vi "Untitled4.vi"() -> ()   [LabVIEW 2024]
uses:
  CANopen Master/CANopen Master.lvclass
  HAL/HAL/Devices/CAN Interfaces/PCAN/PCAN.lvclass
  D:/git/HAL/HAL/Configurations/CFG Base/CFG Base.lvclass
  D:/git/HAL/HAL/Protocols/ICAN/ICAN.lvclass
  CANopen Master/CANopen Master.lvclass/CANopen Master.ctl
  HAL/HAL/Configurations/CFG Base/CFG Base.lvclass
panel:
  in  "Discover Button":bool
  out "Success? DL":bool
  in  "Value":u16
  in  "Multiplexer DL":cluster{"Index":u16, "Sub-Index":u8} {"Index" format="%.0x"}
  in  "Download Button":bool
  in  "Node-ID DL":u8
  out "Available Nodes":map{u8, u8}(c390)
  out "Success? UL":bool
  out "Data UL":u8[](array[numeric]) format="%.0x"
  in  "Node-ID UPL":u8
  in  "Multiplexer":cluster{"Index":u16, "Sub-Index":u8} {"Index" format="%.0x"}
  in  "Upload Button":bool
  out "Emergency?":bool[](array[boolean])
  out "Nodes":u8[](array[numeric])
  in  "stop":bool
  out "Timed Outs?":bool[](array[boolean])
  out "Node-IDs":u8[](array[numeric])
  out "error out":errorcluster
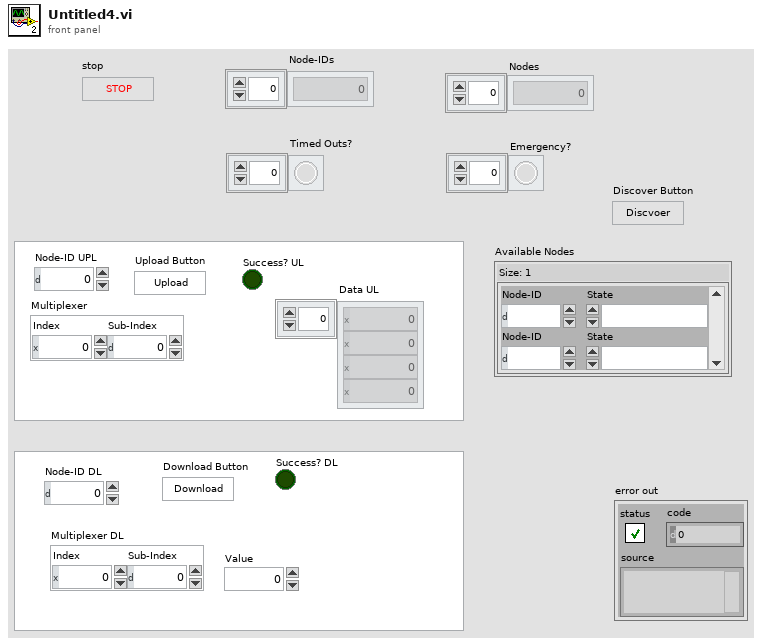
[diagram p1: front panel]
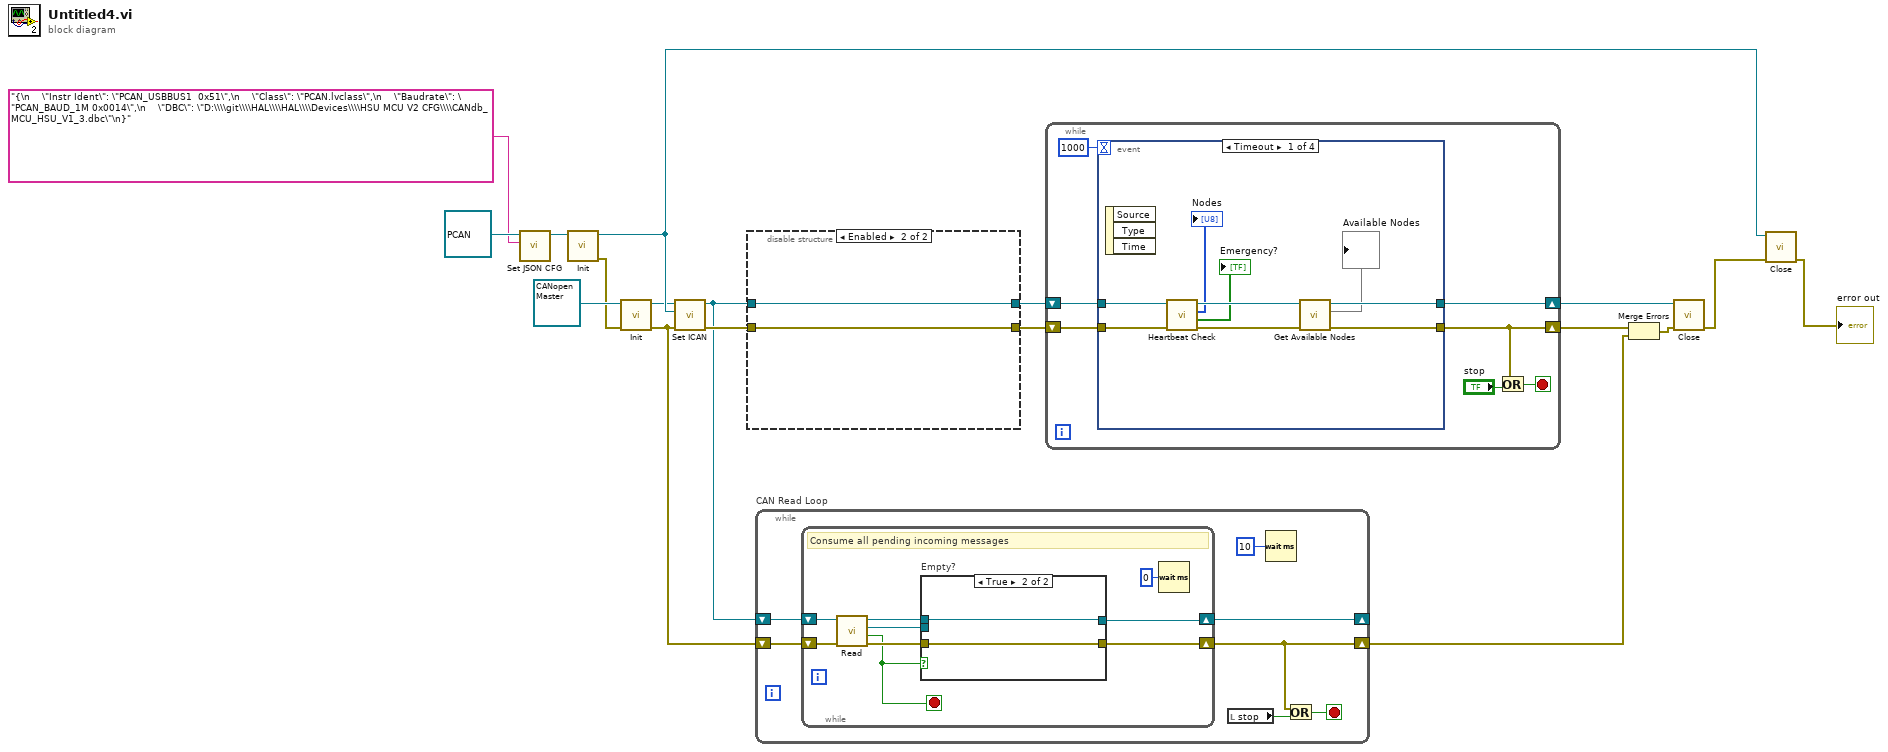
[diagram p0: block diagram]
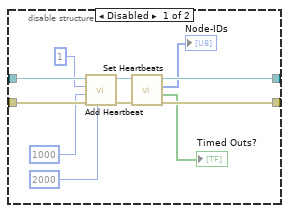
[diagram p2: hidden frame]
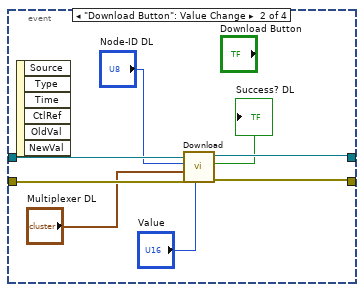
[diagram p3: hidden frame]
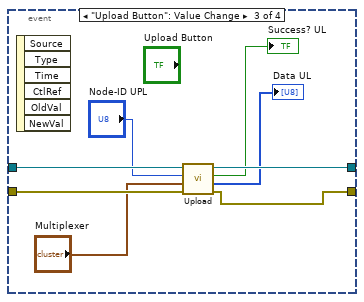
[diagram p4: hidden frame]
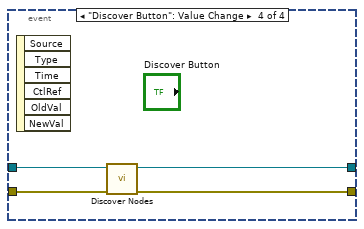
[diagram p5: hidden frame]
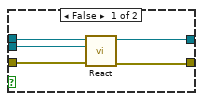
[diagram p6: hidden frame]
diagram:
  n1 = call "Set JSON CFG.vi"("<JSON>CFG"="{\n    \"Instr Ident\": \"PCAN_USBBUS1  0x51\",\n    \"Class\": \"PCAN.lvclass\",\n    \"Baudrate\": \"PCAN_BAUD_1M 0x0014\",\n    \"DBC\": \"D:\\\\git\\\\HAL\\\\HAL\\\\Devices\\\\HSU MCU V2 CFG\\\\CANdb_MCU_HSU_V1_3.dbc\"\n}", "CFG Base in"=refnum<class "PCAN.lvclass"> refnum ("PCAN.lvclass")) -> ("CFG Base out"=w15:refnum<class "PCAN.lvclass">)  [unwired: 9 in]
  n2 = call-dynamic "Init.vi"("PCAN in"=w15) -> ("error out"=w13:errorcluster, "PCAN out"=w12:refnum<class "PCAN.lvclass">)  [unwired: 9 in]
  n3 = call "Init.vi"("error in"=w13, "CANopen Master in"=refnum<class "CANopen Master.lvclass"> refnum ("CANopen Master.lvlib:CANopen Master")) -> ("error out"=w8:errorcluster, "CANopen Master out"=w9:refnum<class "CANopen Master.lvclass">)  [unwired: 8 in]
  n4 = call "Set ICAN.vi"("ICAN"=w12, "CANopen Master in"=w9) -> ("CANopen Master out"=w7:refnum<class "CANopen Master.lvclass">)  [unwired: 9 in]
  n5 = disable-structure shown="Enabled" {
    disable-tunnel: w8 -> [w28 w29]
    disable-tunnel: w7 -> [w27 w30]
    disable-tunnel: [w26 w30] -> w4
    disable-tunnel: [w25 w29] -> w3
    frame Disabled {
      n6 = call "Add Heartbeat.vi"("Timeout"=u16 2000, "error in"=w28, "Period"=u16 1000, "Node-ID"=u8 1, "CANopen Master in"=w27) -> ("error out"=w21:errorcluster, "CANopen Master out"=w20:refnum<class "CANopen Master.lvclass">)  [unwired: 5 in]
      n7 = call "Set Heartbeats.vi"("error in"=w21, "CANopen Master in"=w20) -> ("error out"=w25:errorcluster, "Timed Outs?"=→"Timed Outs?":bool[], "Node-IDs"=→"Node-IDs":u8[], "CANopen Master out"=w26:refnum<class "CANopen Master.lvclass">)  [unwired: 6 in]
    }
    frame Enabled {
    }
  }
  n8 = while "CAN Read Loop" {
    shift-right: [w34] -> w5
    shift-left: w8 -> [w37]
    shift-right: [w33] -> _
    shift-left: w7 -> [w36]
    stop <- w35 stop-if-true
    n9 = while {
      shift-right: [w43] -> w34
      shift-left: w37 -> [w46]
      shift-right: [w39] -> w33
      shift-left: w36 -> [w45]
      stop <- w38 stop-if-true
      # "Consume all pending incoming messages"
      n10 = call "Read.vi"("error in"=w46, "CANopen Master in"=w45) -> ("error out"=w42:errorcluster, "Empty?"=w38:bool, "CANopen Message out"=w44:refnum<class "CANopen Message.lvclass">, "CANopen Master out"=w40:refnum<class "CANopen Master.lvclass">)  [unwired: 6 in]
      n11 = case "Empty?" shown="True" w38 {
        tunnel: w44 -> [w47 _]
        tunnel: [w50 w53] -> w43
        tunnel: w42 -> [w51 w53]
        tunnel: w40 -> [w49 w52]
        tunnel: [w48 w52] -> w39
        frame False {
          n12 = call "React.vi"("error in"=w51, "CANopen Message"=w47, "CANopen Master in"=w49) -> ("error out"=w50:errorcluster, "CANopen Master out"=w48:refnum<class "CANopen Master.lvclass">)  [unwired: 7 in]
        }
        frame True {
        }
      }
      n13 = Wait (ms)(milliseconds to wait=u32 0) -> ()  [unwired: 1 out]
    }
    n14 = local read "stop"() -> (w31:bool)
    n15 = Wait (ms)(milliseconds to wait=10) -> ()  [unwired: 1 out]
    n16 = Or(x=w34, y=w31) -> (x .or. y?=w35:bool)
  }
  n17 = while {
    shift-right: [w57] -> w1
    shift-left: w4 -> [w59]
    shift-right: [w56] -> w2
    shift-left: w3 -> [w58]
    stop <- w55 stop-if-true
    n18 = event shown="[0] Timeout" {
      selector: _ -> [_ _ _ _]
      dyn-events: _ -> [_ _ _ _]
      timeout: 1000 -> [_ _ _ _]
      tunnel: w59 -> [w67 w75 w84 w87]
      tunnel: w58 -> [w68 w76 w83 w88]
      tunnel: [w66 w74 w80 w86] -> w56
      tunnel: [w62 w73 w79 w85] -> w57
      event Timeout {
        n19 = event-data() -> ()  [unwired: 1 in, 3 out]
        n20 = call "Heartbeat Check.vi"("error in"=w68, "CANopen Master in"=w67) -> ("error out"=w66:errorcluster, "Emergency?"=→"Emergency?":bool[], "Nodes"=→"Nodes":u8[], "CANopen Master out"=w65:refnum<class "CANopen Master.lvclass">)  [unwired: 6 in]
        n21 = call "Get Available Nodes.vi"("CANopen Master in"=w65) -> ("Nodes"=→"Available Nodes":map{u8, u8}, "CANopen Master out"=w62:refnum<class "CANopen Master.lvclass">)  [unwired: 8 in, 1 out]
      }
      event "Download Button": Value Change {
        n22 = event-data() -> ()  [unwired: 1 in, 6 out]
        n23 = call "Download.vi"("Value"="Value", "error in"=w76, "Multiplexer"="Multiplexer DL", "Node-ID"="Node-ID DL", "CANopen Master in"=w75) -> ("error out"=w74:errorcluster, "Success?"=→"Success? DL":bool, "CANopen Master out"=w73:refnum<class "CANopen Master.lvclass">)  [unwired: 4 in]
      }
      event "Upload Button": Value Change {
        n24 = event-data() -> ()  [unwired: 1 in, 6 out]
        n25 = call "Upload.vi"("error in"=w83, "Multiplexer"="Multiplexer", "Node-ID"="Node-ID UPL", "CANopen Master in"=w84) -> ("error out"=w80:errorcluster, "Value"=→"Data UL":u8[], "Success?"=→"Success? UL":bool, "CANopen Master out"=w79:refnum<class "CANopen Master.lvclass">)  [unwired: 4 in]
      }
      event "Discover Button": Value Change {
        n26 = event-data() -> ()  [unwired: 1 in, 6 out]
        n27 = call "Discover Nodes.vi"("error in"=w88, "CANopen Master in"=w87) -> ("error out"=w86:errorcluster, "CANopen Master out"=w85:refnum<class "CANopen Master.lvclass">)  [unwired: 8 in]
      }
    }
    n28 = Or(x=w56, y="stop") -> (x .or. y?=w55:bool)
  }
  n29 = Merge Errors(w2, w5) -> (w6:errorcluster)
  n30 = call "Close.vi"("error in"=w6, "CANopen Master in"=w1) -> ("error out"=w11:errorcluster)  [unwired: 8 in, 1 out]
  n31 = call-dynamic "Close.vi"("error in"=w11, "PCAN in"=w12) -> ("error out"=→"error out":errorcluster)  [unwired: 8 in, 1 out]
